vi "Reduce Stock Level.vi"(6 "wait for reply (T)":bool=TRUE, 8 "error in (no error)":errorcluster, 10 "Product":i32) -> (0 "error out":errorcluster, 1 "timed out?":bool, 2 "Reply Payload":T1, 3 "Sucessful?":bool)   [LabVIEW 2019, in "Stock.lvlib"]
doc: "Reduce the stock level and make sure it was sucessful.\n_____\nCreated using Delacor QMH Event Scripter 4.2.1.88."
uses:
  Stock.lvlib
  Reduce Stock Level (Reply Payload)--cluster.ctl
  Reduce Stock Level Argument--cluster.ctl
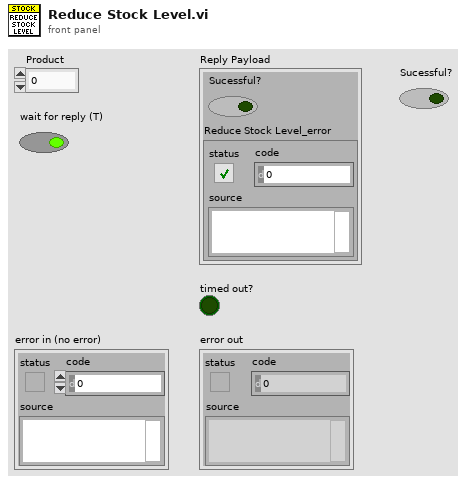
[diagram p1: front panel]
types:
  T1 = typedef "Stock.lvlib/Reduce Stock Level (Reply Payload)--cluster.ctl" = cluster{"Sucessful?":bool, "Reduce Stock Level_error":errorcluster}
  T2 = typedef "Stock.lvlib/Reduce Stock Level Argument--cluster.ctl" = cluster{"Product":i32, "Wait Notifier":refnum<notifier>, "wait for reply":bool}
  T3 = typedef "Stock.lvlib/Request Events--cluster.ctl" = cluster{"Stop Module":refnum<user-event>, "Show Panel":refnum<user-event>, "Hide Panel":refnum<user-event>, "Get Module Execution Status":refnum<user-event>, "Show Diagram":refnum<user-event>, "In Stock and Price":refnum<user-event>, "Reduce Stock Level":refnum<user-event>}
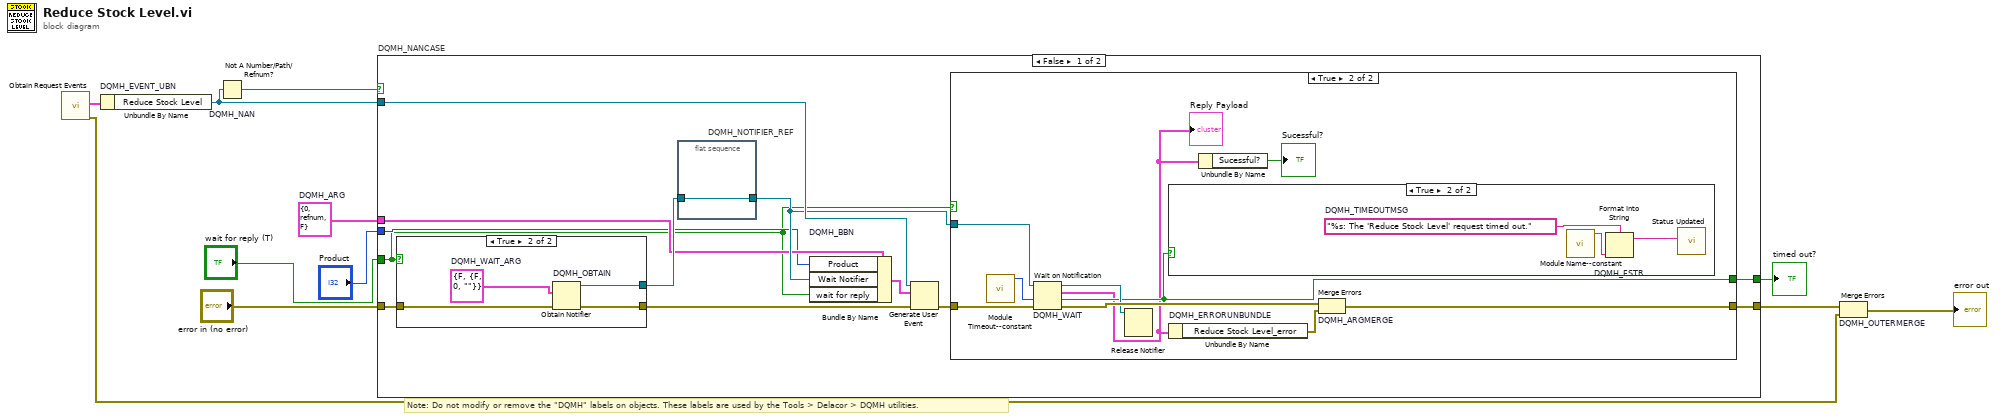
[diagram p0: block diagram]
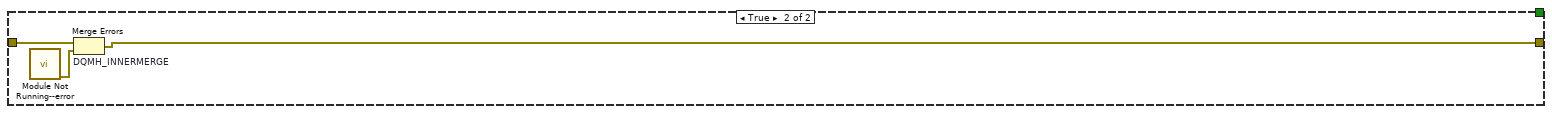
[diagram p5: hidden frame]
diagram:
  w5 = T2 {"Product"=0, "Wait Notifier"=refnum, "wait for reply"=FALSE}  # DQMH_ARG
  # "Note: Do not modify or remove the \"DQMH\" labels on objects. These labels are used by the Tools > Delacor > DQMH utilities."
  n1 = call "Obtain Request Events.vi"() -> ("error out"=w2:errorcluster, "Stock Request Events"=w1:T3)  [unwired: 10 in]
  n2 = Unbundle By Name "DQMH_EVENT_UBN"(w1) -> ("Reduce Stock Level"=w9:refnum<user-event>)
  n3 = Not A Number/Path/Refnum? "DQMH_NAN"(number/path/refnum=w9) -> (NaN/Path/Refnum?=w8:bool)
  n4 = case "DQMH_NANCASE" shown="False" w8 {
    tunnel: "error in (no error)" -> [w23 w46]
    tunnel: w9 -> [w21 _]
    tunnel: [w18 w45] -> w6
    tunnel: [w19 _] -> w7
    tunnel: w5 -> [w14 _]
    tunnel: "Product" -> [w13 _]
    tunnel: "wait for reply (T)" -> [w12 _]
    frame False {
      n5 = case shown="True" w12 {
        tunnel: w23 -> [w39 w43]
        tunnel: [w39 w42] -> w20
        tunnel: [_ w40] -> w16
        frame False {
        }
        frame True {
          w41 = T1 {"Sucessful?"=FALSE, "Reduce Stock Level_error"={"status"=FALSE, "code"=0, "source"=""}}  # DQMH_WAIT_ARG
          n6 = Obtain Notifier "DQMH_OBTAIN"(notification data type=w41, error in (no error)=w43) -> (notifier out=w40:refnum<notifier>, error out=w42:errorcluster)  [unwired: 2 in, 1 out]
        }
      }
      n7 = flat-sequence "DQMH_NOTIFIER_REF" {
        tunnel: w16 -> [w24]
        tunnel: [w24] -> w15
        frame #0 {
        }
      }
      n8 = Bundle By Name "DQMH_BBN"(cluster=w14, "Product"=w13, "Wait Notifier"=w15, "wait for reply"=w12) -> (w17:T2)
      n9 = Generate User Event(user event=w21, event data cluster=w17, error in=w20) -> (error out=w22:errorcluster)  [unwired: 1 in, 1 out]
      n10 = case shown="True" w12 {
        tunnel: w22 -> [w25 w35]
        tunnel: w15 -> [_ w33]
        tunnel: [_ w31] -> w19
        tunnel: [w25 w30] -> w18
        frame False {
        }
        frame True {
          n11 = call "Module Timeout--constant.vi"() -> ("Module Timeout"=w28:i32)  [unwired: 11 in]
          n12 = Wait on Notification "DQMH_WAIT"(notifier=w33, timeout in ms (-1)=w28, error in (no error)=w35) -> (notifier out=w32:refnum<notifier>, notification=w27:T1, timed out?=w31:bool, error out=w34:errorcluster)  [unwired: 1 in]
          "Reply Payload" <- w27
          n13 = Release Notifier(notifier=w32) -> ()  [unwired: 2 in, 3 out]
          n14 = case shown="True" w31 {
            frame False {
            }
            frame True {
              w38 = "%s: The 'Reduce Stock Level' request timed out."  # DQMH_TIMEOUTMSG
              n15 = call "Module Name--constant.vi"() -> ("Module Name"=w37:string)  [unwired: 11 in]
              n16 = Format Into String "DQMH_FSTR"(format string=w38, w37) -> (resulting string=w36:string)  [unwired: 2 in, 1 out]
              n17 = call "Status Updated.vi"("Status"=w36) -> ()  [unwired: 10 in, 1 out]
            }
          }
          n18 = Unbundle By Name "DQMH_ERRORUNBUNDLE"(w27) -> ("Reduce Stock Level_error"=w29:errorcluster)
          n19 = Unbundle By Name(w27) -> ("Sucessful?"=→"Sucessful?":bool)
          n20 = Merge Errors "DQMH_ARGMERGE"(w34, w29) -> (w30:errorcluster)
        }
      }
    }
    frame True {
      n21 = call "Module Not Running--error.vi"() -> ("error out"=w44:errorcluster)  [unwired: 11 in]
      n22 = Merge Errors "DQMH_INNERMERGE"(w46, w44) -> (w45:errorcluster)
    }
  }
  "timed out?" <- w7
  n23 = Merge Errors "DQMH_OUTERMERGE"(w6, w2) -> (→"error out":errorcluster)
